vi "chooseState.vi"(6 "FieldRef":refnum<class "Field.lvclass">, 8 "Robot":refnum<class "Robot.lvclass">, 9 "BallRef":refnum<class "Ball.lvclass">, 10 "OffensiveTeam":refnum<class "Ally.lvclass">, 11 "Utilities in":refnum<class "Utilities.lvclass">) -> (2 "state":T1=enum."GoToReceiveTable")   [LabVIEW 2021]
uses:
  Ball_class/Ball.lvclass
  Ally_class/Ally.lvclass
  D:/RoboIme/horie/SSL_AI/Team_class/Team.lvclass
  Utilities_class/Utilities.lvclass
  Robot_class/Robot.lvclass
  D:/RoboIme/horie/SSL_AI/Object_class/Object.lvclass
  KickToPassReceiverTactic_class/KickToPassReceiverTacticStates.ctl
  Field_class/Field.lvclass
  Robot_class/roles.ctl
  Team_class/Team.lvclass/Team.ctl
  Object_class/Object.lvclass/Object.ctl
  Field_class/Field.lvclass/Field.ctl
  Field_class/Read diagonalLength.vi
  Object_class/Read x.vi
  Object_class/Read y.vi
  Team_class/Read RobotRef.vi
  Team_class/Read OffensivePlay.vi
  <vilib>/Analysis/_algsub.llb/Vector Norm.vi
  <vilib>/Analysis/_algsub.llb/Real Vector Norm.vi
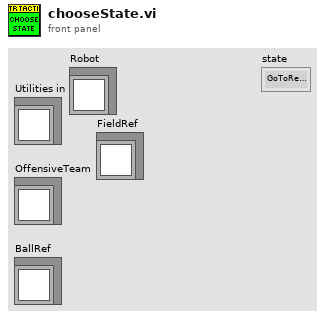
[diagram p1: front panel]
types:
  T1 = typedef "KickToPassReceiverTacticStates.ctl" = enum16{"Halt", "GoToReceiveTable", "KickToPassReceiver", "WaitPass", "Exit"}
  T2 = typedef "roles.ctl" = enum16{"SimpleBallPlacement", "BallPlacementAllyPasser", "BallPlacementAllyReceiver", "BallPlacementEnemy", "5Robots5th", "PassBestReceiver", "5Robots4th", "5Robots3rd", "5Robots2nd", "5Robots1st", "PassBestRobot", "WaitPass", "ABCThirdKicker", "ABCFirstKicker", "ABCSecondKicker", "Tabler", "TableFinalizer", "PrepareRollToPassRoller", "PrepareRollToPassReceiver", "SimplePassRoll", "SimplePassRollReceiver", "PenaltyDefense", "PreparePassReceiver 2", "PreparePassReceiver 1", "PassObserver", "Timeout", "Goto", "ZigZag", "None", "BallOutOfField", "DefenderArea", "Duelist", "AttackerStop", "FollowAttacker", "KeeperRole", "KickPenalty", "AttackerAimGoal", "AttackerBlock", "Marker", "Halt", "Shoot", "PassKicker", "PassReceiver", "TestRole", "PenaltyAttacker"}
  T3 = typedef "OffensivePlay.ctl" = enum16{"5RobotsPassGamePlay", "5PreparePassGame", "5RobotsKeeperGame", "KeeperPassToStriker", "5RobotsNormalGamePlay", "PrepareKeeperPass", "ACBPass", "ABCPass", "PrepareTriplePass", "TableWithStriker", "TableWith2ndStrikerPlay", "PrepareDoublePass", "PrepareRollToPass", "SimplePass", "PreparePass", "PassToStriker", "BallOutOfField", "PassTo2ndStriker", "StopOffensive", "Prepare Penalty Enemy", "EnemyPossessionAtEnemyField", "EnemyPossesionAtOurField", "TestPlay", "PreparePenaltyAlly", "KickPenaltyAlly", "PrepareKickoffAlly", "PrepareKickoffEnemy", "IndirectEnemy", "DirectEnemy", "PreparePassInGame1", "NormalGame", "DirectKick", "Pass", "Halt", "Timeout", "PassPlay", "PenaltyEnemy"}
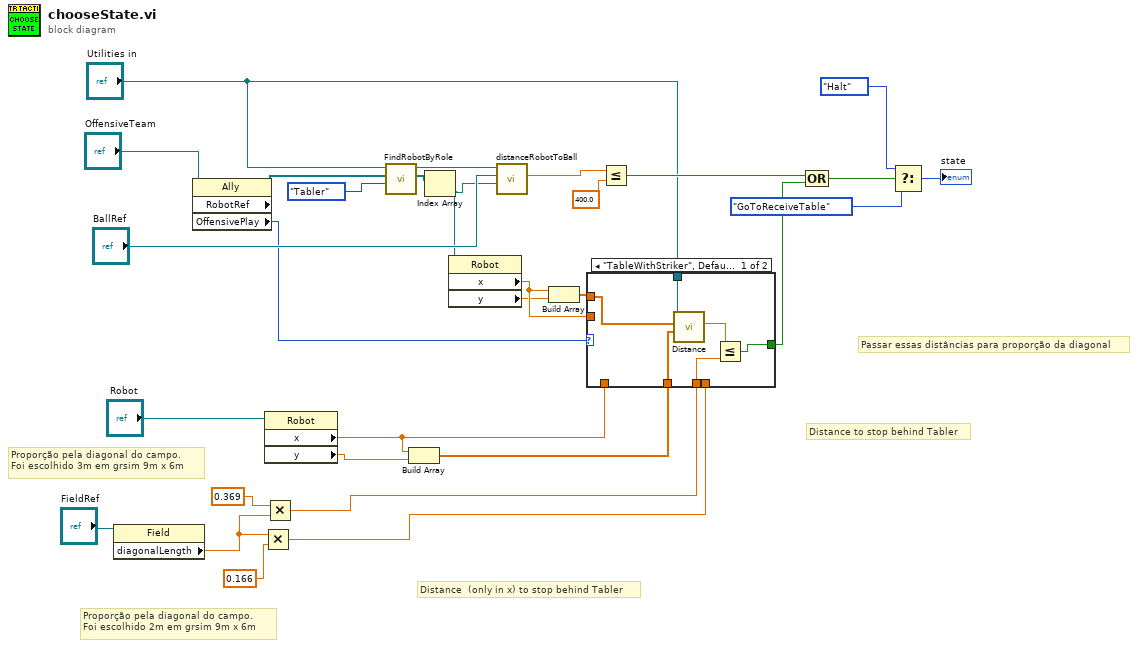
[diagram p0: block diagram]
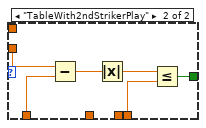
[diagram p2: hidden frame]
diagram:
  # "Proporção pela diagonal do campo.\nFoi escolhido 3m em grsim 9m x 6m"
  # "Proporção pela diagonal do campo.\nFoi escolhido 2m em grsim 9m x 6m"
  # "Passar essas distâncias para proporção da diagonal"
  # "Distance  (only in x) to stop behind Tabler"
  # "Distance to stop behind Tabler"
  n1 = property class="Field"(reference="FieldRef") -> ("diagonalLength"=w1:dbl)  [unwired: 1 in, 2 out]
  n2 = property class="Ally"(reference="OffensiveTeam") -> ("RobotRef"=w24:refnum<class "Robot.lvclass">[], "OffensivePlay"=w21:T3)  [unwired: 1 in, 2 out]
  n3 = Multiply(x=w1, y=0.166) -> (x*y=w4:dbl)
  n4 = property class="Robot"(reference="Robot") -> ("x"=w16:dbl, "y"=w17:dbl)  [unwired: 1 in, 2 out]
  n5 = Multiply(x=0.369, y=w1) -> (x*y=w3:dbl)
  n6 = call "FindRobotByRole.vi"("role"=roles."Tabler", "RobotRef"=w24, "Utilities in"="Utilities in") -> ("Robots"=w27:refnum<class "Robot.lvclass">[], "Utilities out"=w26:refnum<class "Utilities.lvclass">)  [unwired: 6 in, 1 out]
  n7 = Build Array(w16, w17) -> (w15:dbl[])
  n8 = Index Array(array=w27) -> (element=w20:refnum<class "Robot.lvclass">)  [unwired: 1 in]
  n9 = property class="Robot"(reference=w20) -> ("x"=w14:dbl, "y"=w13:dbl)  [unwired: 1 in, 2 out]
  n10 = call "distanceRobotToBall.vi"("Robot"=w20, "Ball"="BallRef", "Utilities in"=w26) -> ("Distance Robot To Ball"=w28:dbl)  [unwired: 6 in, 2 out]
  n11 = Build Array(w14, w13) -> (w12:dbl[])
  n12 = case shown="\"TableWithStriker\", Default" w21 {
    tunnel: [w35 w40] -> w11
    tunnel: w14 -> [_ w39]
    tunnel: w16 -> [_ w38]
    tunnel: w12 -> [w33 _]
    tunnel: w15 -> [w34 _]
    tunnel: "Utilities in" -> [w32 _]
    tunnel: w4 -> [_ w37]
    tunnel: w3 -> [w31 _]
    frame "TableWithStriker", Default {
      n13 = call "Distance.vi"("P1"=w34, "P2"=w33, "Utilities in"=w32) -> ("Distance"=w36:dbl)  [unwired: 6 in, 2 out]
      n14 = Less Or Equal?(x=w36, y=w31) -> (x <= y?=w35:bool)
    }
    frame "TableWith2ndStrikerPlay" {
      n15 = Subtract(x=w39, y=w38) -> (x-y=w42:dbl)
      n16 = Absolute Value(x=w42) -> (abs(x)=w41:dbl)
      n17 = Less Or Equal?(x=w41, y=w37) -> (x <= y?=w40:bool)
    }
  }
  n18 = Less Or Equal?(x=w28, y=400.0) -> (x <= y?=w22:bool)
  n19 = Compound Arithmetic op=OR(w22, w11) -> (w10:bool)
  n20 = Select(t=KickToPassReceiverTacticStates."Halt" ("States"), s=w10, f=KickToPassReceiverTacticStates."GoToReceiveTable" ("States")) -> (s? t:f=→"state":T1)
